vi "Fetch Waveforms.vi"(8 "error in":errorcluster, 11 "IConfigure Scope in":refnum<class "IConfigure Scope.lvclass">) -> (0 "error out":errorcluster, 2 "Last Waveforms":map{u8, waveform(dbl)}(c390), 3 "IConfigure Scope out":refnum<class "IConfigure Scope.lvclass">)   [LabVIEW 2023, in "IConfigure Scope.lvclass"]
uses:
  IConfigure Scope.lvclass
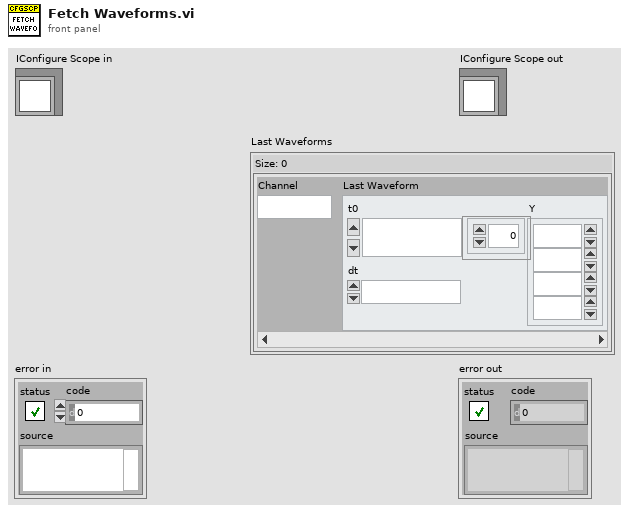
[diagram p1: front panel]
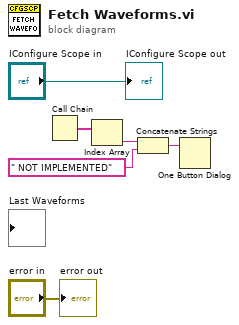
[diagram p0: block diagram]
diagram:
  n1 = Call Chain() -> (call chain=w4:string[])
  n2 = Index Array(array=w4) -> (element=w1:string)  [unwired: 1 in]
  n3 = Concatenate Strings(w1, " NOT IMPLEMENTED" ("string")) -> (w3:string)
  n4 = One Button Dialog(message=w3) -> ()  [unwired: 1 in, 1 out]
  "error out" <- "error in"
  "IConfigure Scope out" <- "IConfigure Scope in"
